vi "Convert XNET to CAN Frame.vi"(11 "XNET frame":T1 {"payload" format="%x"; "timestamp" format="%<%.7X\n%x>T"; "type" items=["CAN Data"=0, "CAN Remote"=1, "CAN Bus Error"=2, "Delay"=224, "Log Trigger"=225, "Start Trigger"=226]; "identifier" format="%x"}) -> (3 "CAN Frame":T3 {"Data" format="%.0x"; "ArbitrationId" format="%.0x"; "Timestamp" format="%<%I:%M:%S%3u %p\n%m/%d/%Y>T"})   [LabVIEW 2013, in "Diagnostics Addon Engine.lvlib"]
uses:
  <vilib>/Automotive Diagnostic Command Set/Diagnostic Transport.llb/Diag CAN Frame Log.ctl
  <vilib>/xnet/xnet.llb/XNET Frame CAN.ctl
  <vilib>/xnet/xnet.llb/XNET Frame Type CAN.ctl
  Diagnostics Addon Engine.lvlib
  <vilib>/addons/Automotive Diagnostic Command Set/NI_Automotive Diagnostic Command Set.lvlib
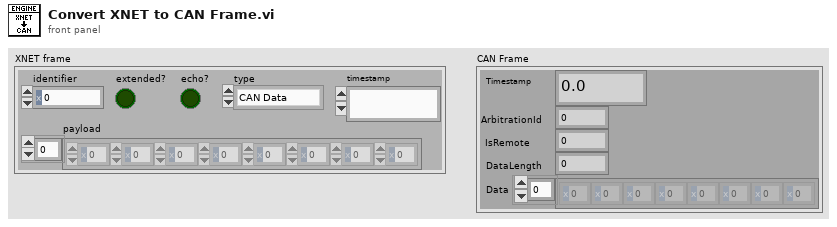
[diagram p1: front panel]
types:
  T1 = typedef "XNET Frame CAN.ctl" = cluster{"timestamp":timestamp, "payload":u8[], "identifier":u32, "type":T2, "extended?":bool, "echo?":bool}
  T2 = typedef "XNET Frame Type CAN.ctl" = u8
  T3 = typedef "NI_Automotive Diagnostic Command Set.lvlib/Diag CAN Frame Log.ctl" = cluster{"Timestamp":dbl, "ArbitrationId":u32, "IsRemote":u8, "DataLength":u8, "Data":u8[]}
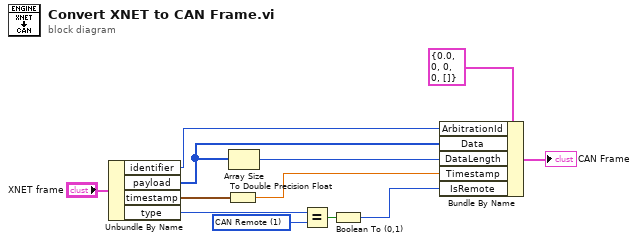
[diagram p0: block diagram]
diagram:
  w3 = T2 1 items=["CAN Data"=0, "CAN Remote"=1, "Delay"=224] ("y")
  n1 = Unbundle By Name("XNET frame") -> ("identifier"=w12:u32, "payload"=w6:u8[], "timestamp"=w8:timestamp, "type"=w4:T2)
  n2 = To Double Precision Float(number=w8) -> (double precision float=w7:dbl)
  n3 = Array Size(array=w6) -> (size(s)=w5:i32)
  n4 = Equal?(x=w4, y=w3) -> (x = y?=w2:bool)
  n5 = Boolean To (0,1)(Boolean=w2) -> (0, 1=w1:i16)
  n6 = Bundle By Name(cluster=T3 {"Timestamp"=0.0, "ArbitrationId"=0, "IsRemote"=0, "DataLength"=0, "Data"=[]} ("element"), "ArbitrationId"=w12, "Data"=w6, "DataLength"=w5, "Timestamp"=w7, "IsRemote"=w1) -> (→"CAN Frame":T3)
